vi "cmd-ack-rebundler.vi"(9 "cmd-response-in":T2, 11 "adam-chassis-cmd-response-in":T3) -> (3 "adam-chassis-cmd-response-out":T3)   [LabVIEW 2020]
uses:
  controls/adam-5000-chassis-cmd-ack.ctl
  controls/adam-5000-cmd-response.ctl
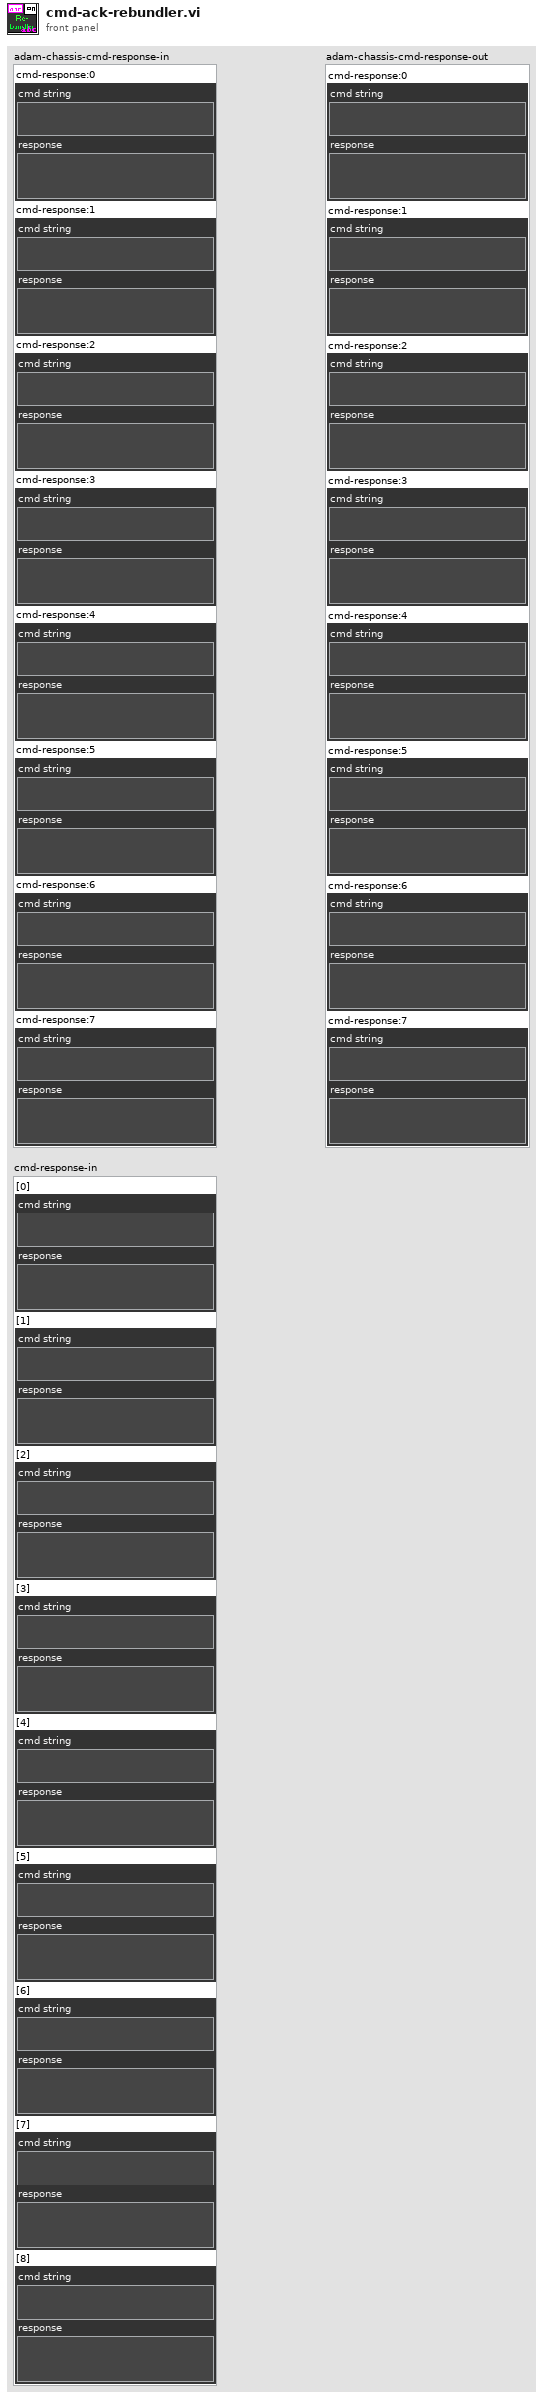
[diagram p1: front panel]
types:
  T1 = typedef "adam-5000-cmd-response.ctl" = cluster{"cmd string":string, "response":string}
  T2 = cluster{"[0]":T1, "[1]":T1, "[2]":T1, "[3]":T1, "[4]":T1, "[5]":T1, "[6]":T1, "[7]":T1, "[8]":T1}
  T3 = typedef "adam-5000-chassis-cmd-ack.ctl" = cluster{"cmd-response:0":T1, "cmd-response:1":T1, "cmd-response:2":T1, "cmd-response:3":T1, "cmd-response:4":T1, "cmd-response:5":T1, "cmd-response:6":T1, "cmd-response:7":T1}
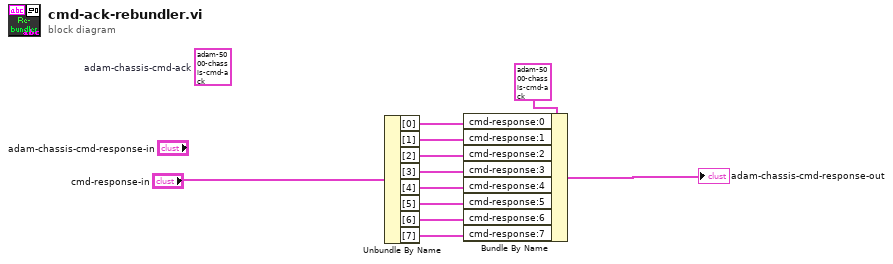
[diagram p0: block diagram]
diagram:
  (unwired) T3 {"cmd-response:0"={"cmd string"="", "response"=""}, "cmd-response:1"={"cmd string"="", "response"=""}, "cmd-response:2"={"cmd string"="", "response"=""}, "cmd-response:3"={"cmd string"="", "response"=""}, "cmd-response:4"={"cmd string"="", "response"=""}, "cmd-response:5"={"cmd string"="", "response"=""}, "cmd-response:6"={"cmd string"="", "response"=""}, "cmd-response:7"={"cmd string"="", "response"=""}}  # adam-chassis-cmd-ack
  n1 = Unbundle By Name("cmd-response-in") -> ("[0]"=w2:T1, "[1]"=w3:T1, "[2]"=w6:T1, "[3]"=w7:T1, "[4]"=w8:T1, "[5]"=w9:T1, "[6]"=w10:T1, "[7]"=w11:T1)
  n2 = Bundle By Name(cluster=T3 {"cmd-response:0"={"cmd string"="", "response"=""}, "cmd-response:1"={"cmd string"="", "response"=""}, "cmd-response:2"={"cmd string"="", "response"=""}, "cmd-response:3"={"cmd string"="", "response"=""}, "cmd-response:4"={"cmd string"="", "response"=""}, "cmd-response:5"={"cmd string"="", "response"=""}, "cmd-response:6"={"cmd string"="", "response"=""}, "cmd-response:7"={"cmd string"="", "response"=""}} ("adam-chassis-cmd-ack"), "cmd-response:0"=w2, "cmd-response:1"=w3, "cmd-response:2"=w6, "cmd-response:3"=w7, "cmd-response:4"=w8, "cmd-response:5"=w9, "cmd-response:6"=w10, "cmd-response:7"=w11) -> (→"adam-chassis-cmd-response-out":T3)
